vi "FTP_DownloadBook.vi"(3 "Parameters":T1={"Book Folder Name"="", "Full file name"="", "Remote Path"="bookfiles/", "Shelf folder"=path "", "Existing books"=[], "Dialog?"=enum."No Dialog", "New Format?"=FALSE}) -> (0 "ZipFile":string, 1 "Parameters":T1={"Book Folder Name"="", "Full file name"="", "Remote Path"="bookfiles/", "Shelf folder"=path "", "Existing books"=[], "Dialog?"=enum."No Dialog", "New Format?"=FALSE})   [LabVIEW 2012]
uses:
  <userlib>/BotSpeak/Devices/EvalRIO/FTPCodes/FTPParameters.ctl
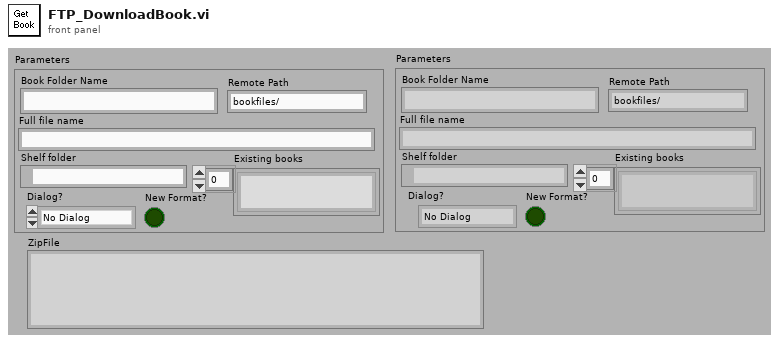
[diagram p1: front panel]
types:
  T1 = typedef "FTPParameters.ctl" = cluster{"Book Folder Name":string, "Full file name":string, "Remote Path":string, "Shelf folder":path, "Existing books":string[], "Dialog?":enum16{"No Dialog", "Dialog", "Overwrite"}, "New Format?":bool}
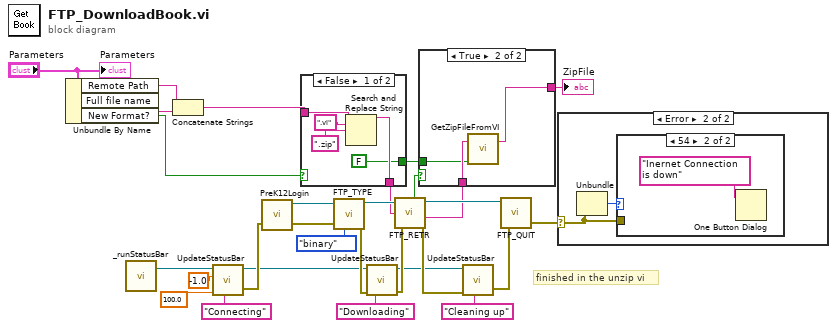
[diagram p0: block diagram]
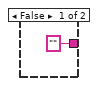
[diagram p2: hidden frame]
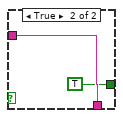
[diagram p3: hidden frame]
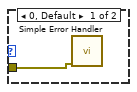
[diagram p5: hidden frame]
diagram:
  # "finished in the unzip vi"
  n1 = Unbundle By Name("Parameters") -> ("Remote Path"=w5:string, "Full file name"=w2:string, "New Format?"=w1:bool)
  n2 = call <userlib>:"_runStatusBar.vi"() -> ("reference out"=w24:refnum<vi>)
  n3 = Concatenate Strings(w5, w2) -> (w9:string)
  n4 = call <userlib>:"UpdateStatusBar.vi"("reference in"=w24, "i"=-1.0, "n"=100.0, "Label"="Connecting") -> ("reference out"=w12:refnum<vi>, "error out"=w22:errorcluster)  [unwired: 1 in]
  n5 = call <userlib>:"PreK12Login.vi"("error in (no error)"=w22) -> ("error out"=w27:errorcluster, "connection ID out"=w26:refnum<k5>)  [unwired: 1 in]
  n6 = case shown="False" w1 {
    tunnel: [w33 w36] -> w10
    tunnel: w9 -> [w34 w36]
    tunnel: [FALSE TRUE] -> w6
    frame False {
      n7 = Search and Replace String(input string=w34, search string=".vi", replace string=".zip" ("search string")) -> (result string=w33:string)  [unwired: 1 in, 7 out]
    }
    frame True {
    }
  }
  n8 = call <userlib>:"FTP_TYPE.vi"("connection ID"=w26, "type (query)"=enum16{"(query)", "ASCII", "binary"}."binary", "error in"=w27) -> ("connection ID out"=w29:refnum<k5>, "error out"=w18:errorcluster)  [unwired: 2 out]
  n9 = call <userlib>:"UpdateStatusBar.vi"("reference in"=w12, "error in (no error)"=w18, "Label"="Downloading") -> ("reference out"=w13:refnum<vi>, "error out"=w17:errorcluster)  [unwired: 2 in]
  n10 = call <userlib>:"FTP_RETR.vi"("connection ID"=w29, "Remote Path"=w10, "error in"=w17) -> ("connection ID out"=w28:refnum<k5>, "vi"=w8:string, "error out"=w15:errorcluster, "Good Reply?"=w7:bool)  [unwired: 1 out]
  n11 = case shown="True" w7 {
    tunnel: w8 -> [_ w40]
    tunnel: w6 -> [_ w39]
    tunnel: ["" ("ZipFile") w38] -> w4
    frame False {
    }
    frame True {
      n12 = call <userlib>:"GetZipFileFromVI.vi"("New Format?"=w39, "VI File"=w40) -> ("ZipFile"=w38:string)  [unwired: 1 out]
    }
  }
  "ZipFile" <- w4
  n13 = call <userlib>:"UpdateStatusBar.vi"("reference in"=w13, "error in (no error)"=w15, "Label"="Cleaning up") -> ("error out"=w14:errorcluster)  [unwired: 2 in, 1 out]
  n14 = call <userlib>:"FTP_QUIT.vi"("connection ID"=w28, "error in"=w14) -> ("error out"=w11:errorcluster)  [unwired: 3 out]
  n15 = case shown="Error" w11 {
    selector: w11 -> [_ w41]
    frame No Error {
    }
    frame Error {
      n16 = Unbundle(w41) -> ("code"=w42:i32)  [unwired: 2 out]
      n17 = case shown="54" w42 {
        tunnel: w41 -> [w43 _]
        frame 0, Default {
          n18 = call <vilib>:"Simple Error Handler.vi"("error in (no error)"=w43) -> ()  [unwired: 1 in, 8 out]
        }
        frame 54 {
          n19 = One Button Dialog(message="Inernet Connection is down") -> ()  [unwired: 2 out]
        }
      }
    }
  }
  "Parameters" <- "Parameters"
